vi "Read Name.vi"(8 "error in (no error)":errorcluster, 11 "Loop in":refnum<class "Loop.lvclass">) -> (0 "error out":errorcluster, 2 "Name":string, 3 "Loop out":refnum<class "Loop.lvclass">)   [LabVIEW 2024, in "Ramses Sequencer.lvlib" / "Loop.lvclass"]
uses:
  Loop.lvclass
  Loop.lvclass/Loop.ctl
  Sequence/Sequence.lvclass
  Base Step/Base Step.lvclass
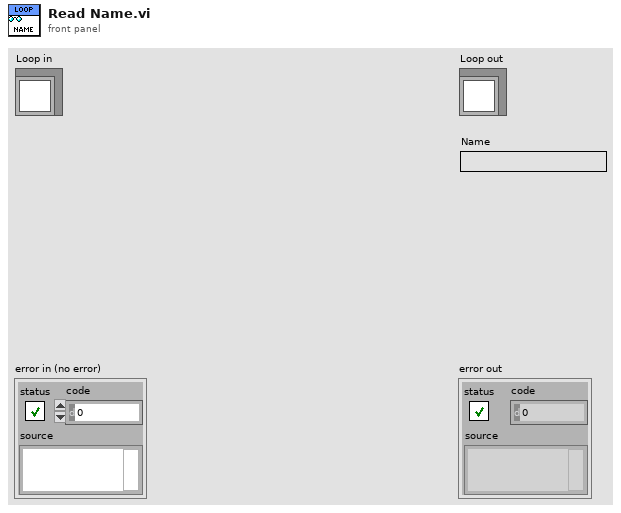
[diagram p1: front panel]
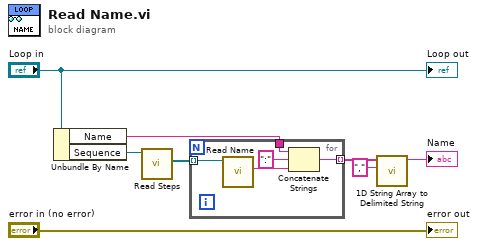
[diagram p0: block diagram]
diagram:
  n1 = Unbundle By Name("Loop in") -> ("Name"=w2:string, "Sequence"=w8:refnum<class "Sequence.lvclass">)
  n2 = call-dynamic "Read Steps.vi"("Sequence in"=w8) -> ("Steps"=w6:refnum<class "Base Step.lvclass">[])  [unwired: 8 in, 2 out]
  n3 = for {
    tunnel: w6 -> [w13] mode=indexing
    tunnel: [w11] -> w4 mode=indexing
    tunnel: w2 -> [w10]
    n4 = call-dynamic "Read Name.vi"("Base Step in"=w13) -> ("Name"=w12:string)  [unwired: 8 in, 2 out]
    n5 = Concatenate Strings(w10, ":" ("string"), w12) -> (w11:string)
  }
  n6 = call <vilib>:"1D String Array to Delimited String.vi"("delimiter"=",", "string array"=w4) -> ("delimited string"=→"Name":string)  [unwired: 9 in]
  "error out" <- "error in (no error)"
  "Loop out" <- "Loop in"
